vi "Read 1 Waveform Channel.vi"() -> ()   [LabVIEW 2020]
uses:
  <instrlib>/LeCroy Wave Series/Public/Data/Read Single Waveform.vi
  <instrlib>/LeCroy Wave Series/LeCroy Wave Series.lvlib
panel:
  in  "Timeout (10000 ms)":u32=10000
  in  "Source (0: Channel 1)":u16(ring) items=["Channel 1", "Channel 2", "Channel 3", "Channel 4", "Memory 1", "Memory 2", "Memory 3", "Memory 4", "Function 1", "Function 2", "Function 3", "Function 4", "Function 5", "Function 6", "Function 7", "Function 8", "Other"]
  out "Waveform Data":waveform(dbl)(graph)
  out "error out":errorcluster
  in  "error in (no error)":errorcluster
  in  "Reset? (T: Yes)":bool=TRUE
  in  "ID Query? (T: Yes)":bool=TRUE
  in  "VISA resource name":refnum<visa-resource-name>
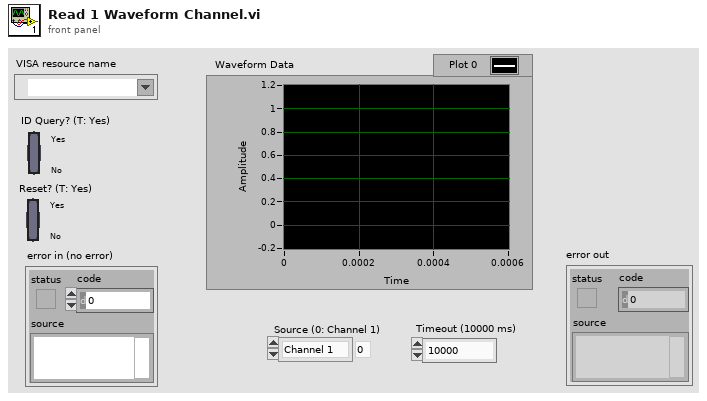
[diagram p1: front panel]
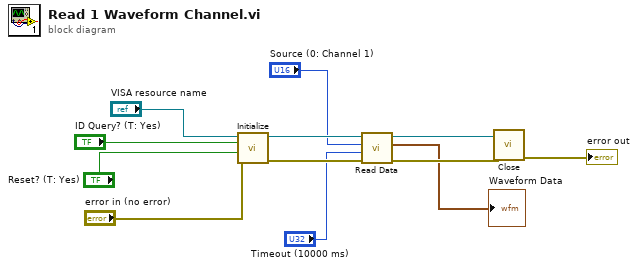
[diagram p0: block diagram]
diagram:
  n1 = call <instrlib>:"Initialize.vi"("error in (no error)"="error in (no error)", "Reset? (T: Yes)"="Reset? (T: Yes)", "ID Query? (T: Yes)"="ID Query? (T: Yes)", "VISA resource name"="VISA resource name") -> ("error out"=w4:errorcluster, "VISA resource name out"=w7:refnum<visa-resource-name>)  [unwired: 6 in]
  n2 = call-poly <instrlib>:"Read Data.vi"("error in (no error)"=w4, "Timeout (10000 ms)"="Timeout (10000 ms)", "Source (0: Channel 1)"="Source (0: Channel 1)", "VISA resource name"=w7) -> ("error out"=w5:errorcluster, "Waveform Data"=→"Waveform Data":waveform(dbl), "VISA resource name out"=w6:refnum<visa-resource-name>)  [unwired: 5 in]
  n3 = call <instrlib>:"Close.vi"("error in (no error)"=w5, "VISA resource name"=w6) -> ("error out"=→"error out":errorcluster)  [unwired: 9 in]
